vi "WFInvertD.vi"(4 "error in (no error)":errorcluster) -> (0 "error out":errorcluster)   [LabVIEW 2013]
panel:
  in  "Waveform In":digitalwaveform(waveform)={"t0"=timestamp(0 s since 1904-01-01), "dt"=1.0, "Y"={"transitions"=[], "data"=[[0, 0, 0, 1], [0, 1, 0, 0]]}}
  out "Waveform Out":digitalwaveform(waveform)={"t0"=timestamp(0 s since 1904-01-01), "dt"=1.0, "Y"={"transitions"=[], "data"=[[0, 0, 0, 1], [0, 1, 0, 0]]}}
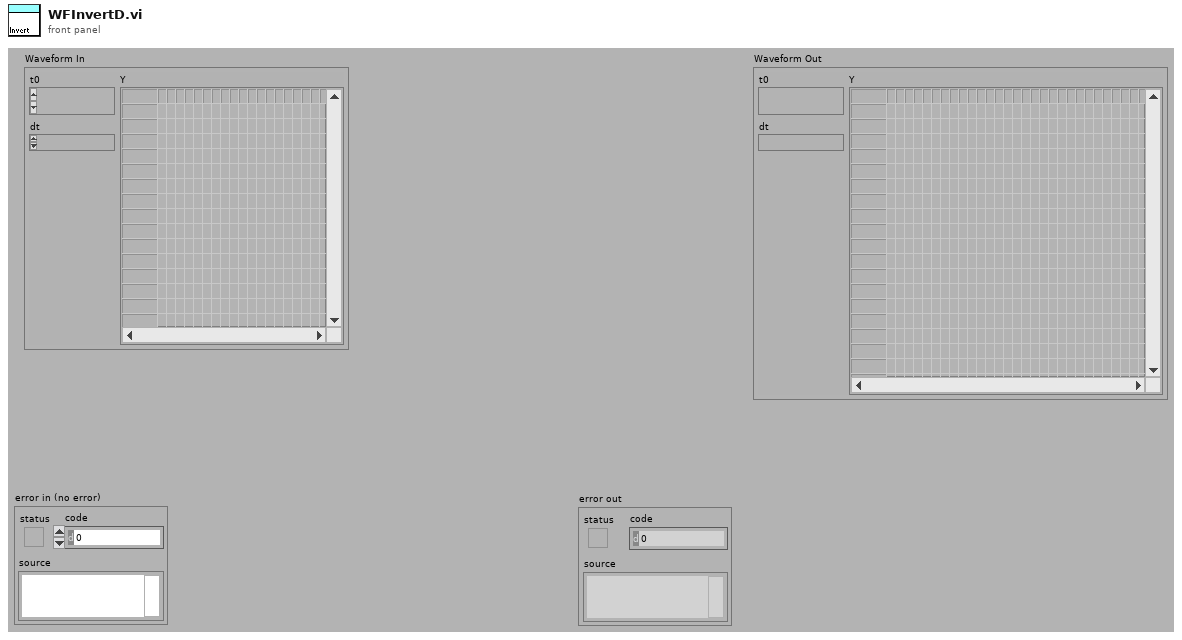
[diagram p1: front panel]
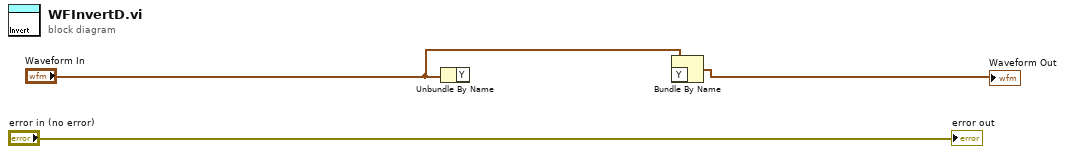
[diagram p0: block diagram]
diagram:
  n1 = Unbundle By Name("Waveform In") -> ("Y"=w1:digitaldata)
  n2 = Bundle By Name(cluster="Waveform In") -> (→"Waveform Out":digitalwaveform)  [unwired: 1 in]
  "error out" <- "error in (no error)"
